vi "destroyFPGA.vi"(8 "error in (no error)":errorcluster, 11 "Boot in":refnum<class "Boot.lvclass">) -> (0 "error out":errorcluster, 3 "Boot out":refnum<class "Boot.lvclass">)   [LabVIEW 2016, in "Boot.lvclass"]
uses:
  Boot.lvclass
  Boot.lvclass/Boot.ctl
  Resources/FPGA/FPGA.lvclass
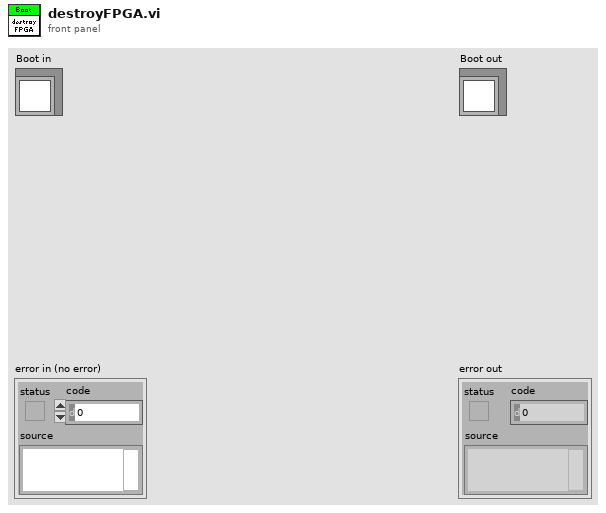
[diagram p1: front panel]
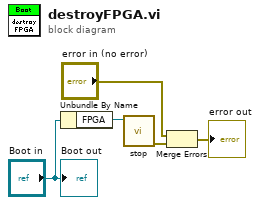
[diagram p0: block diagram]
diagram:
  n1 = Unbundle By Name("Boot in") -> ("FPGA"=w4:refnum<class "FPGA.lvclass">)
  n2 = call "stop.vi"("FPGA in"=w4) -> ("error out"=w3:errorcluster)  [unwired: 9 in, 1 out]
  n3 = Merge Errors("error in (no error)", w3) -> (→"error out":errorcluster)
  "Boot out" <- "Boot in"
